vi "Create.vi"(8 "error in (no error)":errorcluster, 9 "Offset":ext, 10 "Slope":ext) -> (0 "error out":errorcluster, 3 "Trace":refnum<class "Trace.lvclass">)   [LabVIEW 2021, in "Trace.lvclass"]
uses:
  Trace.lvclass
  Trace.lvclass/Trace.ctl
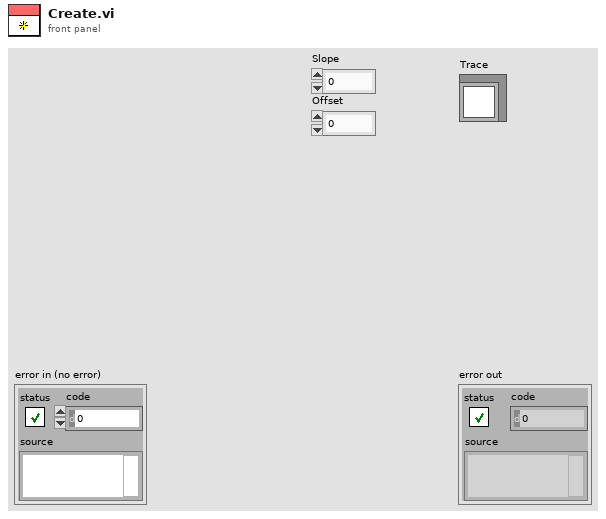
[diagram p1: front panel]
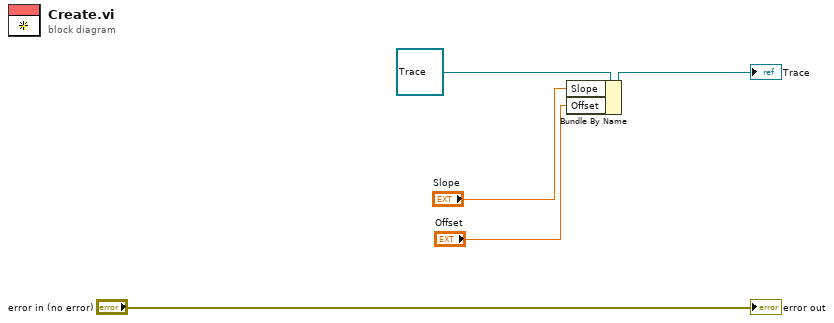
[diagram p0: block diagram]
diagram:
  n1 = Bundle By Name(cluster=refnum<class "Trace.lvclass"> refnum ("Trace"), "Slope"="Slope", "Offset"="Offset") -> (→"Trace":refnum<class "Trace.lvclass">)
  "error out" <- "error in (no error)"
